vi "oax_Save Digital Tacho and Vibration Data.vi"(4 "pulse / rev":i32=1, 5 "reset? (F)":bool, 6 "channel name":string[](array[string]), 7 "channel info":T2[](array[typedef]) {"pregain" format="%.2f"; "weighting filter" items=["Linear", "A-weighting", "B-weighting", "C-weighting", "ITU-R 468-4", "Dolby", "CCITT", "C-message", "Wb", "Wc", "Wd", "We", "Wf", "Wh", "Wj", "Wk", "Wm", "AES17 20 kHz lowpass", "AES17 40 kHz lowpass", "AES17 20 kHz highpass", "AES17 40 kHz highpass"]; "dB reference" format="%^.1e"; "engineering units" items=["custom..."=0, "V"=1, "A"=21, "C"=30, "pC"=31, "s"=32, "-"=29, "Pa"=2, "N"=20, "g"=3, "m/s^2"=4, "m/s"=5, "m"=6, "mm/s"=12, "mm"=13, "micron/s"=14, "micron"=15, "in/s^2"=7, "in/s"=8, "in"=9, "mil/s"=10, "mil"=11, "rad/s^2"=16, "rad/s"=17, "rad"=18, "deg/s^2"=26, "deg/s"=27, "deg"=28, "RPM"=22, "cycle/s^2"=23, "Hz"=24, "cycle"=25, "strain"=19]; "sensor sensitivity" format="%#_5f"}, 8 "error in (no error)":errorcluster, 9 "digital tacho info":T1={"tacho counts"=[], "counter timebase [Hz]"=20000000.0, "counter task type"=enum."event counting", "counter digit (32)"=32}, 10 "waveform data":waveform(dbl)[](array[waveform]), 11 "refnum":refnum<file>) -> (0 "error out":errorcluster, 3 "refnum out":refnum<file>)   [LabVIEW 2017]
doc: "Logs the tachometer and vibration data to a .ddt file."
uses:
  <vilib>/addons/_NISVFA/_Shared subVIs/Controls/svc_Channel Info.ctl
  <vilib>/addons/_NISVFA/_Shared subVIs/Controls/svc_Engineering Units Text Ring.ctl
  <vilib>/addons/_NISVFA/_Shared subVIs/Controls/svc_Weighting Filter Text Ring.ctl
  <vilib>/addons/Sound and Vibration/Order Analysis/Tach Process/SubVIs/digital tach info.ctl
  <vilib>/addons/Sound and Vibration/Order Analysis/Tach Process/SoundVib_TachProcess.lvlib
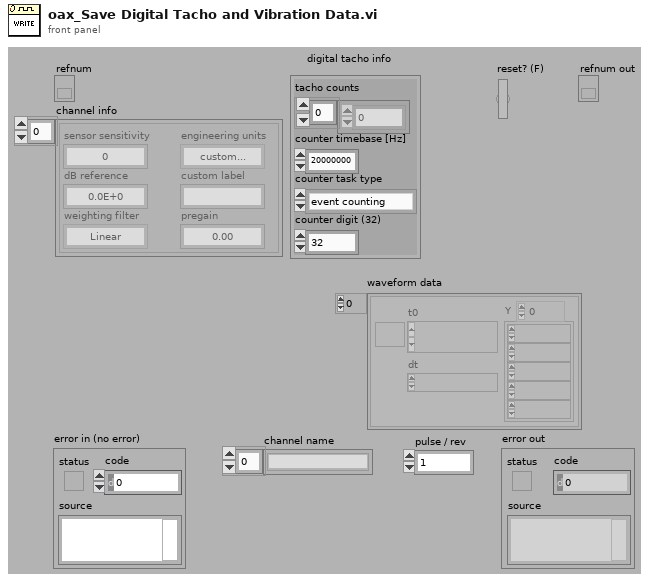
[diagram p1: front panel]
types:
  T1 = typedef "SoundVib_TachProcess.lvlib/digital tach info.ctl" = cluster{"tacho counts":i64[], "counter timebase [Hz]":dbl, "counter task type":enum16{"period measurement", "event counting"}, "counter digit (32)":i32}
  T2 = typedef "svc_Channel Info.ctl" = cluster{"sensor sensitivity":dbl, "engineering units":T3, "dB reference":dbl, "custom label":string, "weighting filter":T4, "pregain":dbl}
  T3 = typedef "svc_Engineering Units Text Ring.ctl" = u16
  T4 = typedef "svc_Weighting Filter Text Ring.ctl" = u16
  T5 = cluster{"digital tacho info":cluster{"tacho counts":i32[], "counter timebase [Hz]":dbl, "counter task type":enum16{"period measurement", "event counting"}, "counter digit (32)":i32}, "waveform data":waveform(dbl)[]}
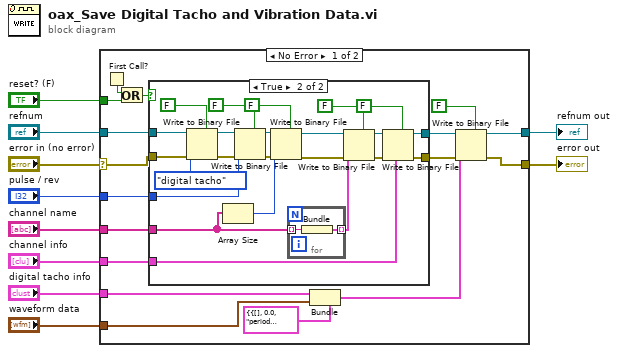
[diagram p0: block diagram]
diagram:
  n1 = case shown="No Error" "error in (no error)" {
    selector: "error in (no error)" -> [w26 w56]
    tunnel: [w16 w56] -> w9
    tunnel: "reset? (F)" -> [w14 _]
    tunnel: "refnum" -> [w27 w55]
    tunnel: "pulse / rev" -> [w25 _]
    tunnel: "channel name" -> [w24 _]
    tunnel: "channel info" -> [w23 _]
    tunnel: "digital tacho info" -> [w22 _]
    tunnel: "waveform data" -> [w21 _]
    tunnel: [w17 w55] -> w1
    frame No Error {
      n2 = First Call?() -> (First Call?: T/F=w12:bool)
      n3 = Or(x=w12, y=w14) -> (x .or. y?=w13:bool)
      n4 = case shown="True" w13 {
        tunnel: w27 -> [w29 w52]
        tunnel: w26 -> [w28 w51]
        tunnel: w25 -> [_ w47]
        tunnel: w24 -> [_ w41]
        tunnel: w23 -> [_ w37]
        tunnel: [w28 w36] -> w20
        tunnel: [w29 w35] -> w19
        frame False {
        }
        frame True {
          n5 = Write to Binary File(file (use dialog)=w52, data=enum16{"analog tacho", "digital tacho"}."digital tacho", error in=w51, 5:FALSE ("prepend array or string size? (T)")) -> (refnum out=w48:refnum<file>, error out=w49:errorcluster)  [unwired: 2 in, 1 out]
          n6 = Array Size(array=w41) -> (size(s)=w44:i32)
          n7 = Write to Binary File(file (use dialog)=w48, data=w47, error in=w49, 5:FALSE ("prepend array or string size? (T)")) -> (refnum out=w45:refnum<file>, error out=w46:errorcluster)  [unwired: 2 in, 1 out]
          n8 = Write to Binary File(file (use dialog)=w45, data=w44, error in=w46, 5:FALSE ("prepend array or string size? (T)")) -> (refnum out=w42:refnum<file>, error out=w43:errorcluster)  [unwired: 2 in, 1 out]
          n9 = for {
            tunnel: w41 -> [w54] mode=indexing
            tunnel: [w53] -> w40 mode=indexing
            n10 = Bundle("ch0 string"=w54) -> (w53:cluster{"ch0 string":string})  [unwired: 1 in]
          }
          n11 = Write to Binary File(file (use dialog)=w42, data=w40, error in=w43, 5:FALSE ("prepend array or string size? (T)")) -> (refnum out=w38:refnum<file>, error out=w39:errorcluster)  [unwired: 2 in, 1 out]
          n12 = Write to Binary File(file (use dialog)=w38, data=w37, error in=w39, 5:FALSE ("prepend array or string size? (T)")) -> (refnum out=w35:refnum<file>, error out=w36:errorcluster)  [unwired: 2 in, 1 out]
        }
      }
      n13 = Bundle(cluster=T5 {"digital tacho info"={"tacho counts"=[], "counter timebase [Hz]"=0.0, "counter task type"=enum."period measurement", "counter digit (32)"=0}, "waveform data"=[]} ("output cluster"), "digital tacho info"=w22, "waveform data"=w21) -> (w18:T5)
      n14 = Write to Binary File(file (use dialog)=w19, data=w18, error in=w20, 5:FALSE ("prepend array or string size? (T)")) -> (refnum out=w17:refnum<file>, error out=w16:errorcluster)  [unwired: 2 in, 1 out]
    }
    frame Error {
    }
  }
  "error out" <- w9
  "refnum out" <- w1
